vi "ChooseSolution.vi"(7 "Solutions":dbl[](array[numeric])) -> (10 "min value":dbl)   [LabVIEW 2011]
panel:
  out "Array":bool[](array[boolean])
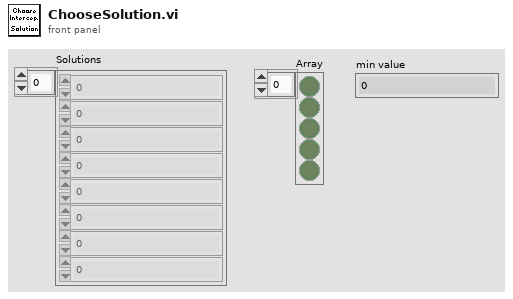
[diagram p1: front panel]
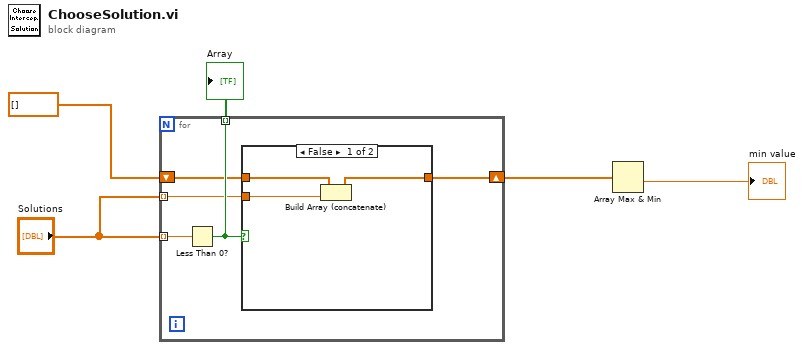
[diagram p0: block diagram]
diagram:
  n1 = for {
    tunnel: "Solutions" -> [w10] mode=indexing
    tunnel: [w9] -> w4 mode=indexing
    tunnel: "Solutions" -> [w8] mode=indexing
    shift-right: [w6] -> w1
    shift-left: dbl[] [] -> [w7]
    n2 = Less Than 0?(x=w10) -> (x < 0?=w9:bool)
    n3 = case shown="False" w9 {
      tunnel: [w11 w14] -> w6
      tunnel: w8 -> [w13 _]
      tunnel: w7 -> [w12 w14]
      frame False {
        n4 = Build Array (concatenate)(w12, w13) -> (w11:dbl[])
      }
      frame True {
      }
    }
  }
  "Array" <- w4
  n5 = Array Max & Min(array=w1) -> (min value=→"min value":dbl)  [unwired: 3 out]
